vi "Configure External Control.vi"(6 "Enable Transient Output (F: False)":bool, 8 "error in (no error)":errorcluster, 9 "Enable Inhibit (F: False)":bool, 10 "External Control (0: Off)":i32(ring) items=["Off", "Level", "Amplifier"], 11 "VISA resource name":refnum<visa-resource-name>) -> (0 "error out":errorcluster, 3 "VISA resource name out":refnum<visa-resource-name>)   [LabVIEW 2015, in "BK Precision 983X Series.lvlib"]
doc: "Configures the external control settings, which include selecting external voltage control or amplifier control mode, and controlling the inhibit and transient state on the digital I/O ports."
uses:
  <instrlib>/BK Precision 983X Series/BK Precision 983X Series.lvlib
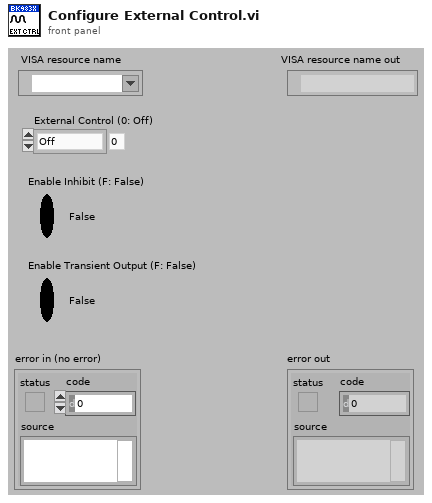
[diagram p1: front panel]
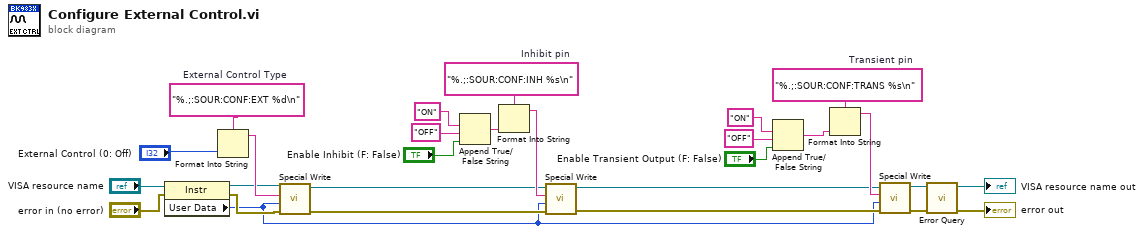
[diagram p0: block diagram]
diagram:
  w10 = "%.;:SOUR:CONF:TRANS %s\n"  # Transient pin
  w25 = "%.;:SOUR:CONF:INH %s\n"  # Inhibit pin
  w26 = "%.;:SOUR:CONF:EXT %d\n"  # External Control Type
  n1 = property class="Instr"(reference="VISA resource name", error in="error in (no error)") -> (reference out=w8:refnum<visa-resource-name>, error out=w7:errorcluster, "User Data"=w1:u32)
  n2 = Format Into String(format string=w26, "External Control (0: Off)") -> (resulting string=w9:string)  [unwired: 2 in, 1 out]
  n3 = call <instrlib>:"Special Write.vi"("error in (no error)"=w7, "Delay (0 ms)"=w1, "Input String"=w9, "VISA resource name"=w8) -> ("error out"=w4:errorcluster, "VISA resource name out"=w5:refnum<visa-resource-name>)  [unwired: 6 in]
  n4 = Append True/False String(1:"Enable Inhibit (F: False)", 2:"OFF", 3:"ON") -> (0:w23:string)  [unwired: 1 in]
  n5 = Format Into String(format string=w25, w23) -> (resulting string=w6:string)  [unwired: 2 in, 1 out]
  n6 = call <instrlib>:"Special Write.vi"("error in (no error)"=w4, "Delay (0 ms)"=w1, "Input String"=w6, "VISA resource name"=w5) -> ("error out"=w2:errorcluster, "VISA resource name out"=w3:refnum<visa-resource-name>)  [unwired: 6 in]
  n7 = Append True/False String(1:"Enable Transient Output (F: False)", 2:"OFF", 3:"ON") -> (0:w20:string)  [unwired: 1 in]
  n8 = Format Into String(format string=w10, w20) -> (resulting string=w13:string)  [unwired: 2 in, 1 out]
  n9 = call <instrlib>:"Special Write.vi"("error in (no error)"=w2, "Delay (0 ms)"=w1, "Input String"=w13, "VISA resource name"=w3) -> ("error out"=w11:errorcluster, "VISA resource name out"=w12:refnum<visa-resource-name>)  [unwired: 6 in]
  n10 = call <instrlib>:"Error Query.vi"("error in (no error)"=w11, "VISA resource name"=w12) -> ("error out"=→"error out":errorcluster, "VISA resource name out"=→"VISA resource name out":refnum<visa-resource-name>)  [unwired: 6 in, 2 out]
